vi "FFT_curve_fit_fcn.vi"(3 "output control":T1, 4 "data":T2, 5 "X":dbl[](array[numeric])) -> (0 "error out":errorcluster, 1 "gradient":dbl[](array[numeric]), 2 "f(X)":dbl)   [LabVIEW 2022 SP3]
doc: "This template is the starting point for creating an objectivel function to be passed to the Unconstrained Optimization.vi."
uses:
  <vilib>/gmath/NumericalOptimization/objective function data.ctl
  Controls/FFT_curve_fit_TD.ctl
  <vilib>/Analysis/NI_AALPro.lvlib
  <vilib>/gmath/NI_Gmath.lvlib
panel:
  in  "Plot?":bool
  out "XY Graph":cluster{"xi used":dbl[], "yi":dbl[]}[](graph)
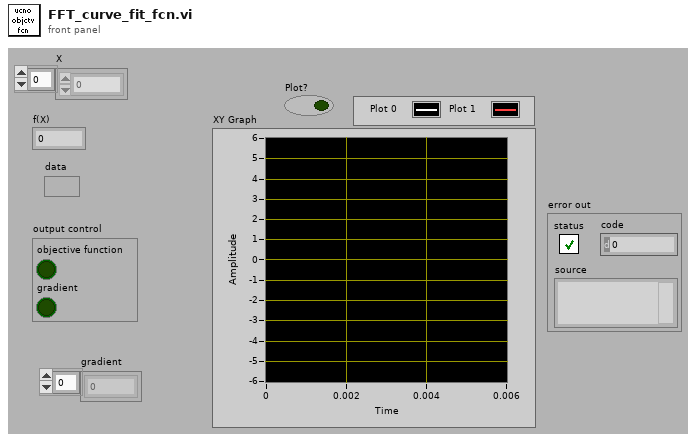
[diagram p1: front panel]
types:
  T1 = cluster{"objective function":bool, "gradient":bool}
  T2 = typedef "NI_Gmath.lvlib/objective function data.ctl" = variant
  T3 = typedef "FFT_curve_fit_TD.ctl" = cluster{"Signal":dbl[], "Frequencies":dbl[], "ti":dbl[], "t":dbl[]}
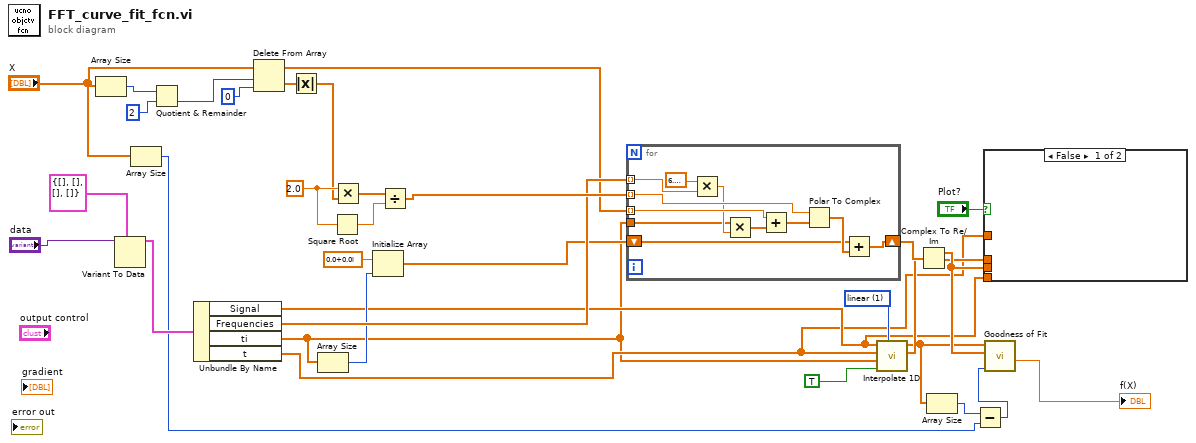
[diagram p0: block diagram]
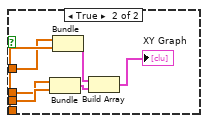
[diagram p2: hidden frame]
diagram:
  w14 = 1 items=["nearest", "linear", "spline", "cubic Hermite", "Lagrange"] ("method")
  w25 = 2.0 ("x")
  n1 = Array Size(array="X") -> (size(s)=w31:i32)
  n2 = Variant To Data(type=T3 {"Signal"=[], "Frequencies"=[], "ti"=[], "t"=[]} ("Cluster"), Variant="data") -> (data=w27:T3)  [unwired: 1 in, 1 out]
  n3 = Array Size(array="X") -> (size(s)=w10:i32)
  n4 = Quotient & Remainder(x=w31, y=2) -> (floor(x/y)=w29:i32)  [unwired: 1 out]
  n5 = Unbundle By Name(w27) -> ("Signal"=w5:dbl[], "Frequencies"=w21:dbl[], "ti"=w3:dbl[], "t"=w4:dbl[])
  n6 = Delete From Array(array="X", length=w29, index=0) -> (deleted portion=w23:dbl[], array with subset deleted=w20:dbl[])
  n7 = Absolute Value(x=w23) -> (abs(x)=w1:dbl[])
  n8 = Array Size(array=w3) -> (size(s)=w18:i32)
  n9 = Square Root(x=w25) -> (sqrt(x)=w24:dbl)
  n10 = Multiply(x=w25, y=w1) -> (x*y=w26:dbl[])
  n11 = Initialize Array(cdb 0.0+0.0i ("element"), w18) -> (w17:cdb[])
  n12 = Divide(x=w26, y=w24) -> (x/y=w22:dbl[])
  n13 = for {
    tunnel: w22 -> [w42] mode=indexing
    tunnel: w20 -> [w44] mode=indexing
    tunnel: w3 -> [w38]
    tunnel: w21 -> [w41] mode=indexing
    shift-right: [w36] -> w15
    shift-left: w17 -> [w34]
    n14 = Multiply(x=6.283185307179586, y=w41) -> (x*y=w39:dbl)
    n15 = Multiply(x=w38, y=w39) -> (x*y=w37:dbl[])
    n16 = Add(x=w44, y=w37) -> (x+y=w43:dbl[])
    n17 = Polar To Complex(1:w43, 2:w42) -> (0:w35:cdb[])
    n18 = Add(x=w34, y=w35) -> (x+y=w36:cdb[])
  }
  n19 = call <vilib>:"Interpolate 1D.vi"("method"=w14, "X is monotonic"=TRUE, "xi"=w3, "X"=w4, "Y"=w5) -> ("xi used"=w7:dbl[], "yi"=w6:dbl[])  [unwired: 4 in, 1 out]
  n20 = Complex To Re/Im(x + iy=w15) -> (x=w8:dbl[])  [unwired: 1 out]
  n21 = Array Size(array=w6) -> (size(s)=w12:i32)
  n22 = Subtract(x=w12, y=w10) -> (x-y=w9:i32)
  n23 = case shown="False" "Plot?" {
    tunnel: w8 -> [_ w51]
    tunnel: w7 -> [_ w50]
    tunnel: w5 -> [_ w46]
    tunnel: w4 -> [_ w45]
    frame False {
    }
    frame True {
      n24 = Bundle("xi used"=w50, w51) -> (w48:cluster{"xi used":dbl[], dbl[]})  [unwired: 1 in]
      n25 = Bundle("t"=w45, "Signal"=w46) -> (w49:cluster{"t":dbl[], "Signal":dbl[]})  [unwired: 1 in]
      n26 = Build Array(w49, w48) -> (→"XY Graph":cluster{"xi used":dbl[], "Signal":dbl[]}[])
    }
  }
  n27 = call <vilib>:"Goodness of Fit.vi"("degree of freedom"=w9, "Best Fit"=w8, "Y"=w6) -> ("RMSE"=→"f(X)":dbl)  [unwired: 5 in, 3 out]
